vi "TestLevelProbe.vi"() -> ()   [LabVIEW 2018]
panel:
  out "read buffer":string
  in  "stop":bool
  out "error out":errorcluster
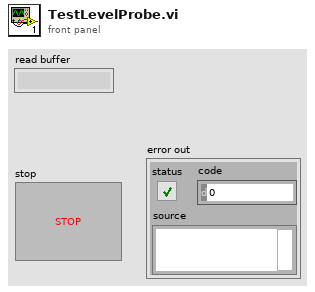
[diagram p1: front panel]
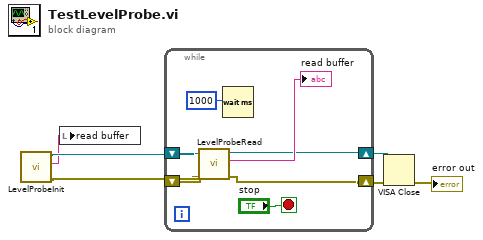
[diagram p0: block diagram]
diagram:
  n1 = call "LevelProbeInit.vi"() -> ("error out"=w3:errorcluster, "read buffer"=w1:string, "VISA resource name out"=w2:refnum<visa-resource-name>)  [unwired: 9 in]
  n2 = local write "read buffer"(w1) -> ()
  n3 = while {
    shift-right: [w8] -> w6
    shift-left: w2 -> [w11]
    shift-right: [w7] -> w5
    shift-left: w3 -> [w10]
    stop <- "stop" stop-if-true
    n4 = call "LevelProbeRead.vi"("error in"=w10, "VISA resource name"=w11) -> ("error out"=w7:errorcluster, "read buffer"=→"read buffer":string, "VISA resource name out"=w8:refnum<visa-resource-name>)  [unwired: 6 in, 1 out]
    n5 = Wait (ms)(milliseconds to wait=1000) -> ()  [unwired: 1 out]
  }
  n6 = VISA Close(VISA resource name=w6, error in (no error)=w5) -> (error out=→"error out":errorcluster)
